vi "UtilityLib.get command line parameters.vi"(8 "error in (no error)":errorcluster) -> (0 "error out":errorcluster, 1 "parametersOriginal":string[](array[string]), 2 "parametersCleaned":string[](array[string]))   [LabVIEW 2014, in "UtilityLib.lvlib"]
doc: "Gets the command line parameters of THIS application. Remark: This routine tries to solve the problem of the ever changing numbering of command line paramters passed to LabVIEW."
uses:
  UtilityLib.lvlib
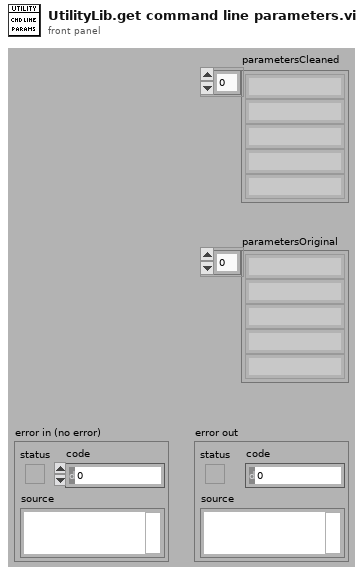
[diagram p1: front panel]
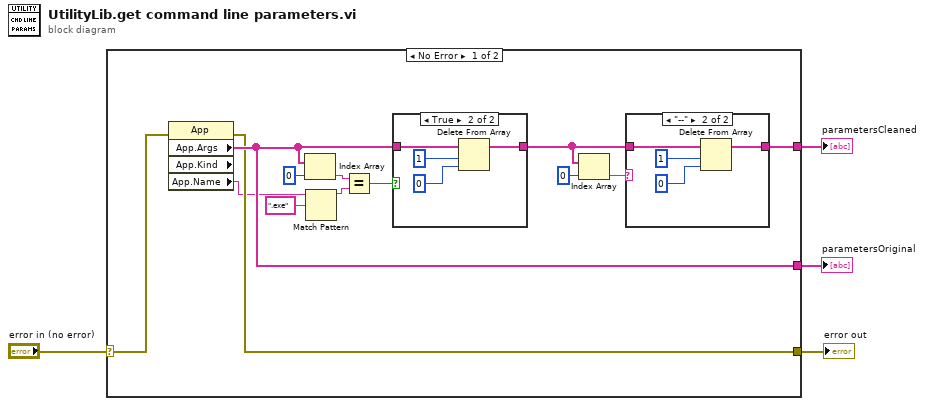
[diagram p0: block diagram]
diagram:
  n1 = case shown="No Error" "error in (no error)" {
    selector: "error in (no error)" -> [w11 w28]
    tunnel: [w17 _] -> w4
    tunnel: [w13 _] -> w3
    tunnel: [w12 w28] -> w2
    frame No Error {
      n2 = property class="App" props=["App.Args", "App.Kind", "App.Name"](error in=w11) -> (error out=w12:errorcluster, "App.Args"=w17:string[], "App.Name"=w9:string)  [unwired: 1 in, 2 out]
      n3 = Index Array(array=w17, index=0) -> (element=w6:string)
      n4 = Match Pattern(string=w9, regular expression=".exe") -> (before substring=w5:string)  [unwired: 1 in, 3 out]
      n5 = Equal?(x=w6, y=w5) -> (x = y?=w7:bool)
      n6 = case shown="True" w7 {
        tunnel: w17 -> [w18 w22]
        tunnel: [w18 w21] -> w14
        frame False {
        }
        frame True {
          n7 = Delete From Array(array=w22, length=1, index=0) -> (array with subset deleted=w21:string[])  [unwired: 1 out]
        }
      }
      n8 = Index Array(array=w14, index=0) -> (element=w16:string)
      n9 = case shown="\"--\"" w16 {
        tunnel: w14 -> [w23 w27]
        tunnel: [w23 w26] -> w13
        frame Default {
        }
        frame "--" {
          n10 = Delete From Array(array=w27, length=1, index=0) -> (array with subset deleted=w26:string[])  [unwired: 1 out]
        }
      }
    }
    frame Error {
    }
  }
  "parametersCleaned" <- w3
  "parametersOriginal" <- w4
  "error out" <- w2
